vi "Remote Module DataSocket Decorator.vi"() -> ()   [LabVIEW 2019]
uses:
  <extravilib>/ChannelInstances/Event Messenger-c(str,var)/Instantiate.vi
  <extravilib>/ChannelInstances/Event Messenger-c(str,var)/))Channel.vi
  <extravilib>/ChannelInstances/Event Messenger-c(str,var).lvlib
panel:
  out "error out":errorcluster
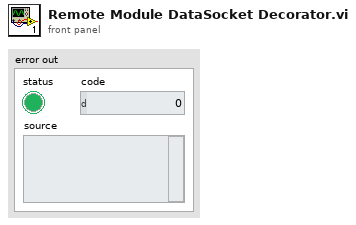
[diagram p1: front panel]
types:
  T1 = enum16{"Read", "Write", "ReadWrite", "BufferedRead", "BufferedReadWrite"}
  T2 = typedef "Event Messenger-c(str,var).lvlib/))Channel.ctl" = refnum<queue>
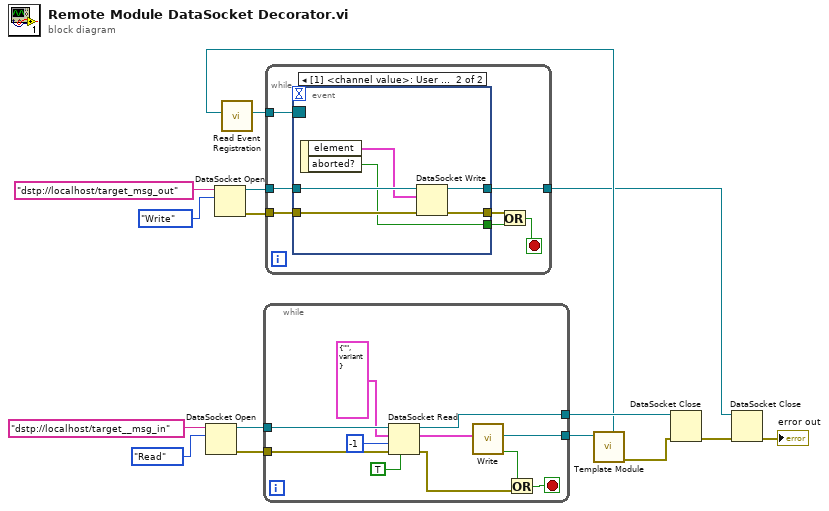
[diagram p0: block diagram]
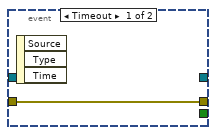
[diagram p2: hidden frame]
diagram:
  n1 = DataSocket Open(10:T1."Read" ("mode"), 11:"dstp://localhost/target__msg_in" ("URL")) -> (0:w16:errorcluster, 3:w15:refnum<k13>)  [unwired: 2 in]
  n2 = DataSocket Open(10:T1."Write" ("mode"), 11:"dstp://localhost/target_msg_out" ("URL")) -> (0:w6:errorcluster, 3:w7:refnum<k13>)  [unwired: 2 in]
  n3 = while {
    tunnel: w16 -> [w27]
    tunnel: w15 -> [w26]
    tunnel: [w22] -> w11
    tunnel: [w21] -> w10
    stop <- w18 stop-if-true
    n4 = DataSocket Read(6:TRUE ("wait for updated value (T)"), 8:w27, 9:-1 ("ms timeout (10000)"), 10:cluster{"cmd":string, "data":variant} {"cmd"="", "data"=variant} ("message"), 11:w26) -> (0:w19:errorcluster, 2:w20:cluster{"cmd":string, "data":variant}, 3:w22:refnum<k13>)  [unwired: 4 out]
    n5 = call <extravilib>:"Write.vi"("element"=w20) -> ("done?"=w17:bool, "channel"=w21:T2)  [unwired: 9 in]
    n6 = Or(x=w17, y=w19) -> (x .or. y?=w18:bool)
  }
  n7 = call "Template Module.vi"("Message Input"=w10) -> ("error out"=w12:errorcluster, "Message Output"=w5:T2)  [unwired: 9 in]
  n8 = call <extravilib>:"Read Event Registration.vi"("channel"=w5) -> ("event registration refnum"=w2:refnum<event-registration>)  [unwired: 10 in]
  n9 = while {
    tunnel: w6 -> [w32]
    tunnel: w7 -> [w33]
    tunnel: w2 -> [w34]
    tunnel: [w31] -> w1
    stop <- w29 stop-if-true
    n10 = event shown="[1] <channel value>: User Event" {
      selector: w34 -> [_ _]
      dyn-events: _ -> [_ _]
      timeout: _ -> [_ _]
      tunnel: w33 -> [_ w40]
      tunnel: w32 -> [w35 w41]
      tunnel: [_ w38] -> w31
      tunnel: [w35 w37] -> w30
      tunnel: [_ w36] -> w28
      event Timeout {
        n11 = event-data() -> ()  [unwired: 1 in, 3 out]
      }
      event User Event {
        n12 = event-data() -> ("element"=w39:cluster{"cmd":string, "data":variant}, "aborted?"=w36:bool)  [unwired: 1 in]
        n13 = DataSocket Write(8:w41, 10:w39, 11:w40) -> (0:w37:errorcluster, 3:w38:refnum<k13>)  [unwired: 1 in, 1 out]
      }
    }
    n14 = Or(x=w30, y=w28) -> (x .or. y?=w29:bool)
  }
  n15 = DataSocket Close(8:w12, 11:w11) -> (0:w4:errorcluster)  [unwired: 1 in, 1 out]
  n16 = DataSocket Close(8:w4, 11:w1) -> (0:→"error out":errorcluster)  [unwired: 1 in, 1 out]
